vi "Arduino角度.vi"(4 "error in":errorcluster, 5 "read buffer":string) -> (1 "error out":errorcluster, 2 "Waveform Chart":cluster{dbl, dbl}(graph))   [LabVIEW 2017]
panel:
  out "Y":dbl
  out "X":dbl
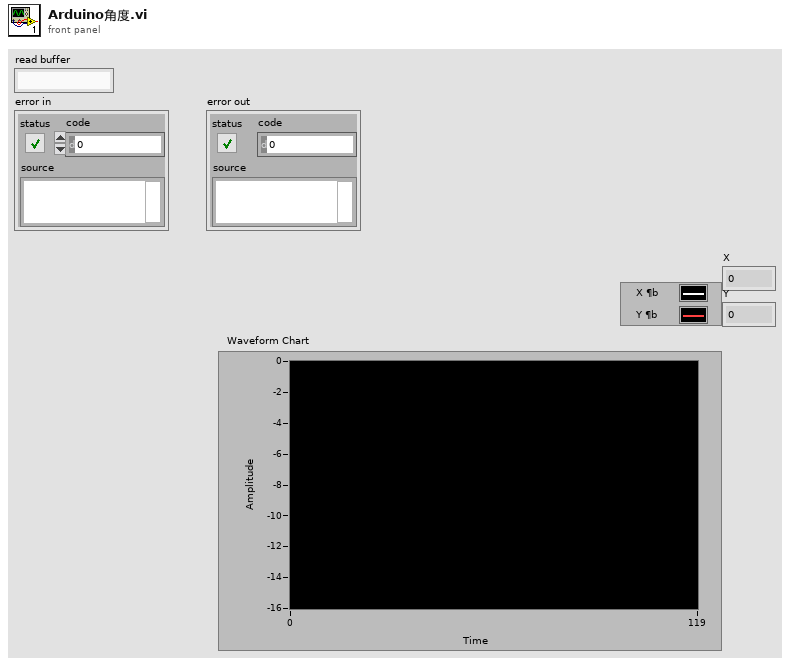
[diagram p1: front panel]
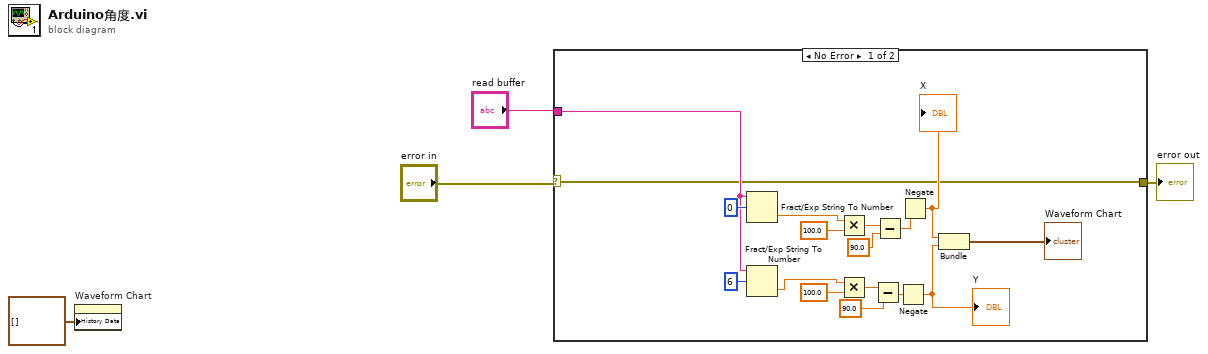
[diagram p0: block diagram]
diagram:
  n1 = property on="Waveform Chart" class="WFChart (strict)"("History Data"=cluster{dbl, dbl}[] []) -> ()  [unwired: 2 in, 2 out]
  n2 = case shown="No Error" "error in" {
    selector: "error in" -> [w7 w22]
    tunnel: [w7 w22] -> w1
    tunnel: "read buffer" -> [w8 _]
    frame No Error {
      n3 = Fract/Exp String To Number(string=w8, offset=0) -> (number=w16:dbl)  [unwired: 2 in, 1 out]
      n4 = Fract/Exp String To Number(string=w8, offset=6) -> (number=w15:dbl)  [unwired: 2 in, 1 out]
      n5 = Multiply(x=w16, y=100.0) -> (x*y=w21:dbl)
      n6 = Multiply(x=w15, y=100.0) -> (x*y=w20:dbl)
      n7 = Subtract(x=w20, y=90.0) -> (x-y=w6:dbl)
      n8 = Subtract(x=w21, y=90.0) -> (x-y=w10:dbl)
      n9 = Negate(x=w6) -> (-x=w5:dbl)
      "Y" <- w5
      n10 = Negate(x=w10) -> (-x=w9:dbl)
      "X" <- w9
      n11 = Bundle(w9, w5) -> (→"Waveform Chart":cluster{dbl, dbl})  [unwired: 1 in]
    }
    frame Error {
    }
  }
  "error out" <- w1
